vi "Settings_FGV.vi"(8 "error in (no error)":errorcluster, 11 "State":enum16{"Get_settings", "Set_settings"}(ring)) -> (0 "error out":errorcluster, 3 "Settings":T1)   [LabVIEW 2012]
uses:
  controls/Video_analizer_settings.ctl
  <vilib>/Utility/config.llb/Read Key (Double).vi
  <vilib>/Utility/config.llb/Write Key (Double).vi
  <vilib>/Utility/config.llb/Write Key (Boolean).vi
  <vilib>/Utility/config.llb/Write Key (U32).vi
  <vilib>/Utility/config.llb/NI_LVConfig.lvlib
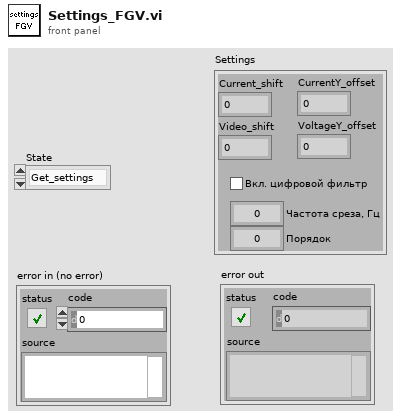
[diagram p1: front panel]
types:
  T1 = typedef "Video_analizer_settings.ctl" = cluster{"Current_shift":dbl, "Video_shift":dbl, "CurrentY_offset":dbl, "VoltageY_offset":dbl, "FIR_enable":bool, "Cutof_freq":dbl, "Order":u32}
  T2 = enum32{"invalid app kind", "Development System", "Run Time System", "Student Edition", "Embedded LabVIEW", "Evaluation", "Custom"}
  T3 = typedef "NI_LVConfig.lvlib/Config Data RefNum.ctl" = refnum<k1>
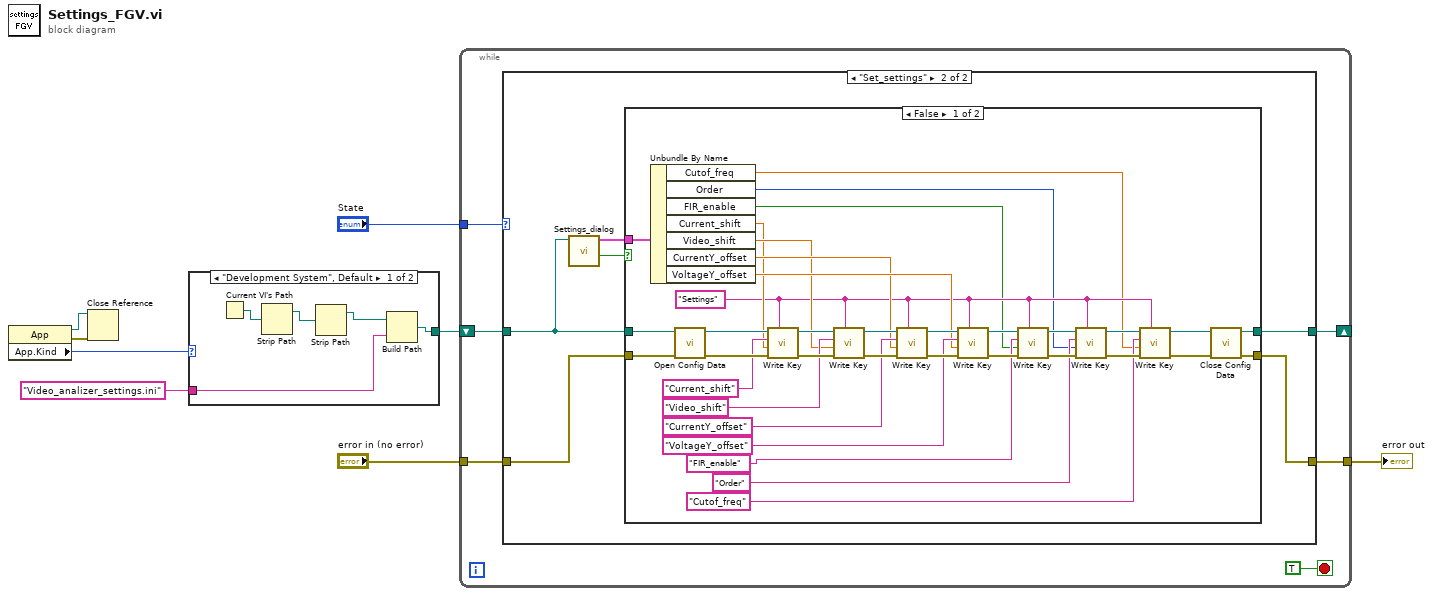
[diagram p0: block diagram]
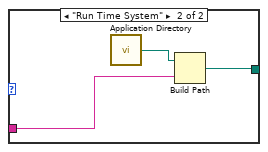
[diagram p2: hidden frame]
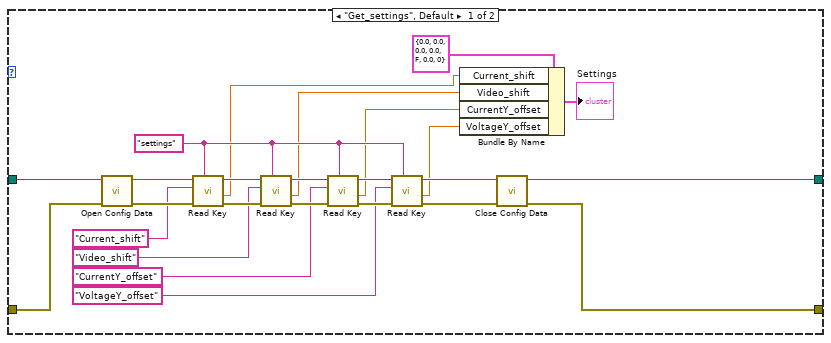
[diagram p3: hidden frame]
diagram:
  n1 = property class="App"() -> (reference out=w4:refnum<vi>, error out=w5:errorcluster, "App.Kind"=w3:T2)  [unwired: 2 in]
  n2 = Close Reference(reference=w4, error in (no error)=w5) -> ()  [unwired: 1 out]
  n3 = case shown="\"Development System\", Default" w3 {
    tunnel: [w11 w15] -> w2
    tunnel: "Video_analizer_settings.ini" ("name or relative path") -> [w12 w14]
    frame "Development System", Default {
      n4 = Current VI's Path() -> (path=w13:path)
      n5 = Strip Path(path=w13) -> (stripped path=w10:path)  [unwired: 1 out]
      n6 = Strip Path(path=w10) -> (stripped path=w9:path)  [unwired: 1 out]
      n7 = Build Path(base path=w9, name or relative path=w12) -> (appended path=w11:path)
    }
    frame "Run Time System" {
      n8 = call <vilib>:"Application Directory.vi"() -> ("Application Directory"=w16:path)
      n9 = Build Path(base path=w16, name or relative path=w14) -> (appended path=w15:path)
    }
  }
  n10 = while {
    tunnel: "State" -> [w21]
    tunnel: "error in (no error)" -> [w20]
    tunnel: [w19] -> w6
    shift-right: [w18] -> _
    shift-left: w2 -> [w17]
    stop <- TRUE stop-if-true
    n11 = case shown="\"Set_settings\"" w21 {
      tunnel: w20 -> [w41 w53]
      tunnel: [w40 w52] -> w19
      tunnel: [w42 w51] -> w18
      tunnel: w17 -> [w45 w48]
      frame "Get_settings", Default {
        w33 = "settings" ("section")
        n12 = call <vilib>:"Open Config Data.vi"("error in (no error)"=w41, "configuration file path"=w45) -> ("error out"=w44:errorcluster, "refnum"=w43:T3)  [unwired: 7 in, 1 out]
        n13 = call-poly <vilib>:"Read Key.vi"("section"=w33, "error in (no error)"=w44, "key"="Current_shift", "refnum"=w43) -> ("error out"=w46:errorcluster, "value"=w26:dbl, "refnum out"=w47:T3)  [unwired: 4 in, 1 out]
        n14 = call-poly <vilib>:"Read Key.vi"("section"=w33, "error in (no error)"=w46, "key"="Video_shift", "refnum"=w47) -> ("error out"=w39:errorcluster, "value"=w25:dbl, "refnum out"=w36:T3)  [unwired: 4 in, 1 out]
        n15 = call-poly <vilib>:"Read Key.vi"("section"=w33, "error in (no error)"=w39, "key"="CurrentY_offset", "refnum"=w36) -> ("error out"=w38:errorcluster, "value"=w24:dbl, "refnum out"=w35:T3)  [unwired: 4 in, 1 out]
        n16 = call-poly <vilib>:"Read Key.vi"("section"=w33, "error in (no error)"=w38, "key"="VoltageY_offset", "refnum"=w35) -> ("error out"=w37:errorcluster, "value"=w23:dbl, "refnum out"=w34:T3)  [unwired: 4 in, 1 out]
        n17 = Bundle By Name(cluster=T1 {"Current_shift"=0.0, "Video_shift"=0.0, "CurrentY_offset"=0.0, "VoltageY_offset"=0.0, "FIR_enable"=FALSE, "Cutof_freq"=0.0, "Order"=0} ("Settings"), "Current_shift"=w26, "Video_shift"=w25, "CurrentY_offset"=w24, "VoltageY_offset"=w23) -> (→"Settings":T1)
        n18 = call <vilib>:"Close Config Data.vi"("error in (no error)"=w37, "refnum"=w34) -> ("error out"=w40:errorcluster, "file path"=w42:path)  [unwired: 8 in]
      }
      frame "Set_settings" {
        n19 = call "Settings_dialog.vi"("Initial_cofig"=w48) -> ("canceled or no change?"=w50:bool, "Settings"=w49:T1)  [unwired: 9 in]
        n20 = case shown="False" w50 {
          tunnel: w53 -> [w89 w90]
          tunnel: [w88 w90] -> w52
          tunnel: [w87 w91] -> w51
          tunnel: w48 -> [w86 w91]
          tunnel: w49 -> [w73 _]
          frame False {
            w60 = "Settings" ("section")
            n21 = Unbundle By Name(w73) -> ("Cutof_freq"=w54:dbl, "Order"=w55:u32, "FIR_enable"=w56:bool, "Current_shift"=w69:dbl, "Video_shift"=w70:dbl, "CurrentY_offset"=w71:dbl, "VoltageY_offset"=w72:dbl)
            n22 = call <vilib>:"Open Config Data.vi"("error in (no error)"=w89, "configuration file path"=w86) -> ("error out"=w85:errorcluster, "refnum"=w83:T3)  [unwired: 7 in, 1 out]
            n23 = call-poly <vilib>:"Write Key.vi"("section"=w60, "error in (no error)"=w85, "value"=w69, "key"="Current_shift", "refnum"=w83) -> ("error out"=w84:errorcluster, "refnum out"=w82:T3)  [unwired: 4 in, 1 out]
            n24 = call-poly <vilib>:"Write Key.vi"("section"=w60, "error in (no error)"=w84, "value"=w70, "key"="Video_shift", "refnum"=w82) -> ("error out"=w79:errorcluster, "refnum out"=w77:T3)  [unwired: 4 in, 1 out]
            n25 = call-poly <vilib>:"Write Key.vi"("section"=w60, "error in (no error)"=w79, "value"=w71, "key"="CurrentY_offset", "refnum"=w77) -> ("error out"=w78:errorcluster, "refnum out"=w76:T3)  [unwired: 4 in, 1 out]
            n26 = call-poly <vilib>:"Write Key.vi"("section"=w60, "error in (no error)"=w78, "value"=w72, "key"="VoltageY_offset", "refnum"=w76) -> ("error out"=w68:errorcluster, "refnum out"=w64:T3)  [unwired: 4 in, 1 out]
            n27 = call-poly <vilib>:"Write Key.vi"("section"=w60, "error in (no error)"=w68, "value"=w56, "key"="FIR_enable", "refnum"=w64) -> ("error out"=w67:errorcluster, "refnum out"=w63:T3)  [unwired: 4 in, 1 out]
            n28 = call-poly <vilib>:"Write Key.vi"("section"=w60, "error in (no error)"=w67, "value"=w55, "key"="Order", "refnum"=w63) -> ("error out"=w66:errorcluster, "refnum out"=w62:T3)  [unwired: 4 in, 1 out]
            n29 = call-poly <vilib>:"Write Key.vi"("section"=w60, "error in (no error)"=w66, "value"=w54, "key"="Cutof_freq", "refnum"=w62) -> ("error out"=w65:errorcluster, "refnum out"=w61:T3)  [unwired: 4 in, 1 out]
            n30 = call <vilib>:"Close Config Data.vi"("error in (no error)"=w65, "refnum"=w61) -> ("error out"=w88:errorcluster, "file path"=w87:path)  [unwired: 8 in]
          }
          frame True {
          }
        }
      }
    }
  }
  "error out" <- w6
